vi "CreateWhitelist.vi"(8 "error in (no error)":errorcluster) -> (0 "error out":errorcluster, 3 "Whitelist out":refnum<class "Whitelist.lvclass">)   [LabVIEW 2019, in "Whitelist.lvclass"]
doc: "Creates a new whitelist."
uses:
  Whitelist.lvclass
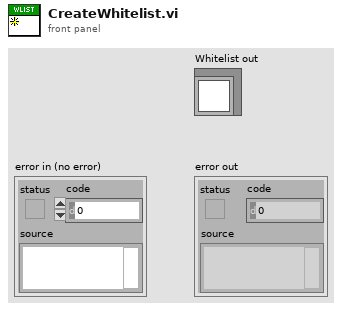
[diagram p1: front panel]
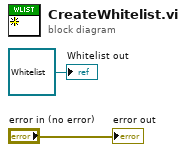
[diagram p0: block diagram]
diagram:
  "error out" <- "error in (no error)"
  "Whitelist out" <- refnum<class "Whitelist.lvclass"> refnum ("Whitelist in")
